vi "Feedback Evaporative Cooler Demo.vi"() -> ()   [LabVIEW 2015]
uses:
  Cooler/Cooler/Cooler.lvclass
  Cooler UI/Cooler Panel/Cooler Panel.lvclass
  <vilib>/ActorFramework/Message Enqueuer/Message Enqueuer.lvclass/Message Enqueuer.ctl
  <vilib>/ActorFramework/Message Enqueuer/Enqueue.vi
  <vilib>/ActorFramework/Message Priority Queue/Priority Enqueue.vi
  <vilib>/ActorFramework/Stop Msg/Stop Msg.lvclass
  <vilib>/ActorFramework/Actor/Actor.lvclass
panel:
  in  "Bouton Stop":bool
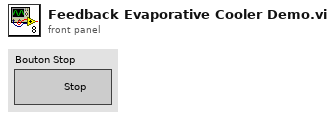
[diagram p1: front panel]
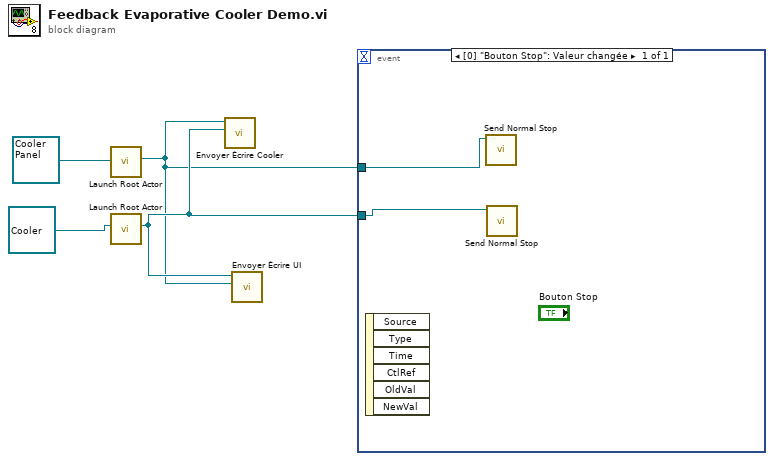
[diagram p0: block diagram]
diagram:
  n1 = call <vilib>:"Launch Root Actor.vi"("Actor"=refnum<class "Cooler Panel.lvclass"> refnum ("Cooler UI.lvlib:Cooler Panel.lvclass")) -> ("Actor's Enqueuer"=w1:refnum<class "Message Enqueuer.lvclass">)  [unwired: 9 in, 1 out]
  n2 = call <vilib>:"Launch Root Actor.vi"("Actor"=refnum<class "Cooler.lvclass"> refnum ("Cooler.lvlib:Cooler.lvclass")) -> ("Actor's Enqueuer"=w2:refnum<class "Message Enqueuer.lvclass">)  [unwired: 9 in, 1 out]
  n3 = call "Envoyer Écrire Cooler.vi"("Framework d'acteur:Objet ajoutant des msgs à la file"=w2, "Message Enqueuer"=w1) -> ()  [unwired: 8 in, 2 out]
  n4 = call "Envoyer Écrire UI.vi"("Framework d'acteur:Objet ajoutant des msgs à la file"=w1, "Message Enqueuer"=w2) -> ()  [unwired: 8 in, 2 out]
  n5 = event shown="[0] \"Bouton Stop\": Valeur changée" {
    selector: _ -> [_]
    dyn-events: _ -> [_]
    timeout: _ -> [_]
    tunnel: w1 -> [w6]
    tunnel: w2 -> [w5]
    event "Bouton Stop": Value Change {
      n6 = event-data() -> ()  [unwired: 1 in, 6 out]
      n7 = call <vilib>:"Send Normal Stop.vi"("Message Enqueuer"=w6) -> ()  [unwired: 10 in, 1 out]
      n8 = call <vilib>:"Send Normal Stop.vi"("Message Enqueuer"=w5) -> ()  [unwired: 10 in, 1 out]
    }
  }
